vi "dfd_Map Win Const.vi"(1 "new window (8.0)":u16(ring)=9 items=["None"=0, "Hanning"=1, "Hamming"=2, "Blackman-Harris"=3, "Exact Blackman"=4, "Blackman"=5, "Flat Top"=6, "4 Term B-Harris"=7, "7 Term B-Harris"=8, "Low Sidelobe"=9, "Triangular"=30, "Kaiser"=60, "Dolph-Chebyshev"=61]) -> (0 "old window (7.0)":T1(ring))   [LabVIEW 2017, in "NI_DigFilter_Design.lvlib"]
uses:
  <vilib>/addons/Digital Filter Design/NI_DigFilter_Design.lvlib
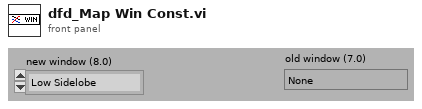
[diagram p1: front panel]
types:
  T1 = enum16{"None ", "Hanning", "Hamming", "Blackman-Harris", "Exact Blackman", "Blackman", "Flat Top", "4 Term B-Harris ", "7 Term B-Harris", "Low Sidelobe"}
  T2 = enum16{"None ", "Hanning", "Hamming", "Blackman-Harris", "Exact Blackman", "Blackman", "Flat Top", "4 Term B-Harris ", "7 Term B-Harris", "Low Sidelobe"}[]
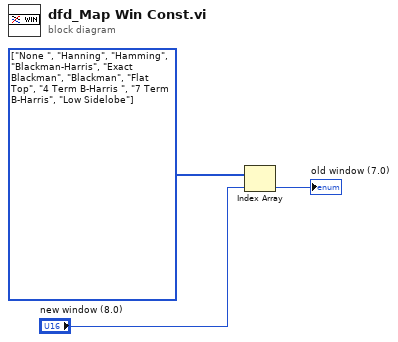
[diagram p0: block diagram]
diagram:
  w3 = T2 [enum."None ", enum."Hanning", enum."Hamming", enum."Blackman-Harris", enum."Exact Blackman", enum."Blackman", enum."Flat Top", enum."4 Term B-Harris ", enum."7 Term B-Harris", enum."Low Sidelobe"] items=["None ", "Hanning", "Hamming", "Blackman-Harris", "Exact Blackman", "Blackman", "Flat Top", "4 Term B-Harris ", "7 Term B-Harris", "Low Sidelobe"] ("appended array")
  n1 = Index Array(array=w3, index="new window (8.0)") -> (element=→"old window (7.0)":T1)
